vi "calc_phase_map.vi"(3 "noise threshold":dbl=20.0, 4 "u8_ar_image_pixel_array":dbl[][][](array[numeric]), 5 "image name":string="fringe") -> (0 "raw phase map array":dbl[][](array[numeric]), 2 "phase map":T1(plugin-control))   [LabVIEW 2011]
uses:
  global_vars.vi
panel:
  in  "add":dbl
  in  "multi":dbl
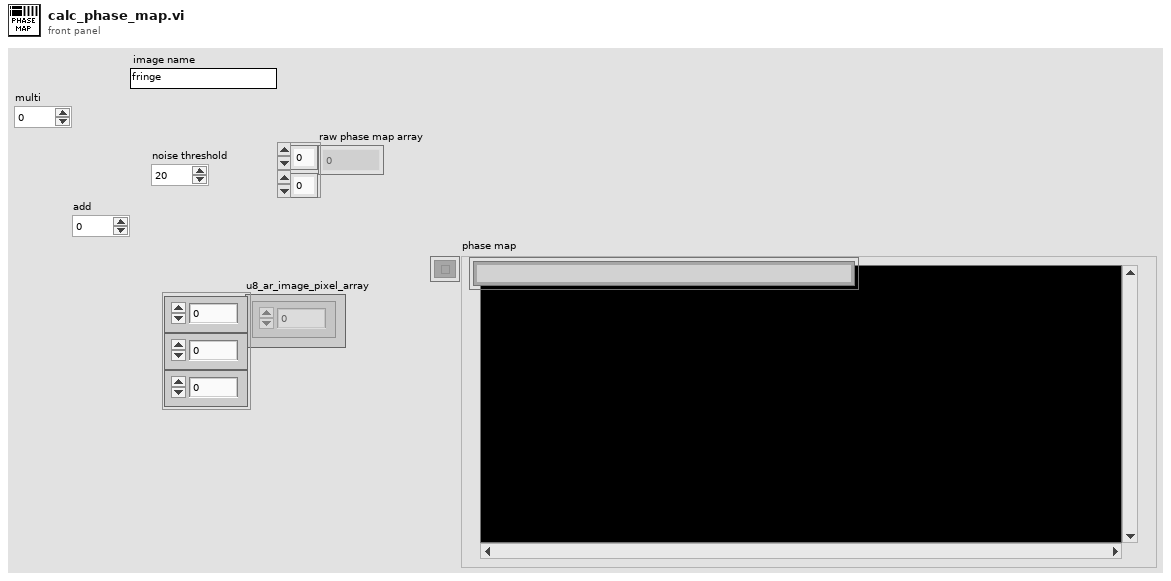
[diagram p1: front panel]
types:
  T1 = typedef "IMAQ Image.ctl" = refnum<image>
  T2 = typedef "Image Type" = u32
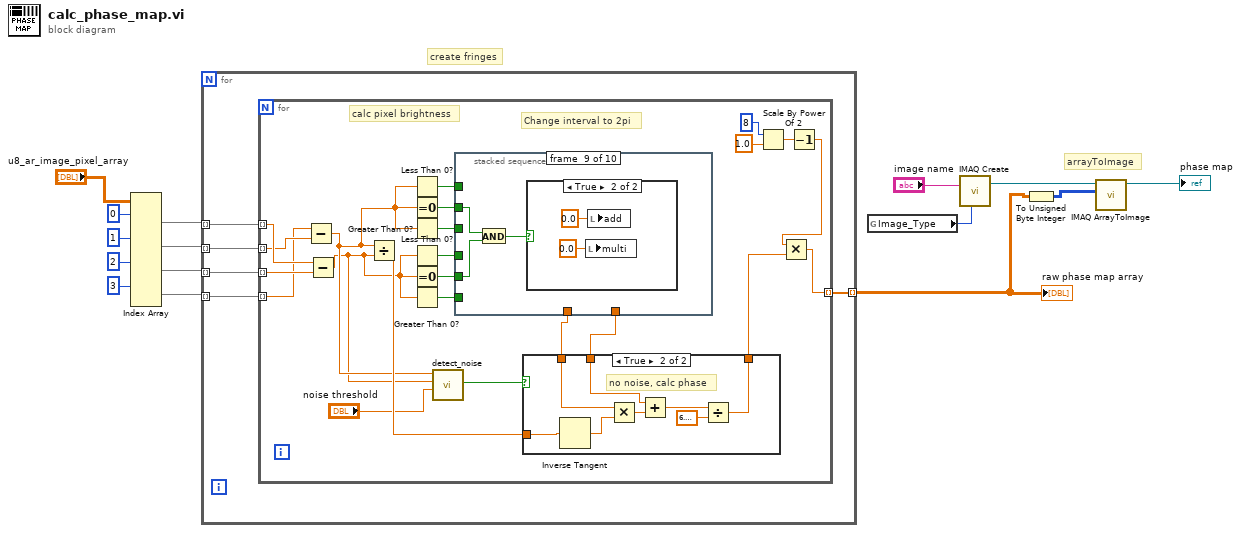
[diagram p0: block diagram]
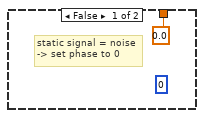
[diagram p2: hidden frame]
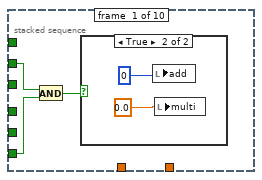
[diagram p3: hidden frame]
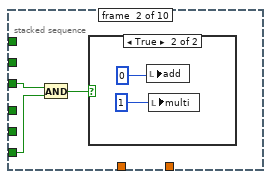
[diagram p5: hidden frame]
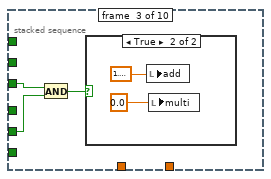
[diagram p7: hidden frame]
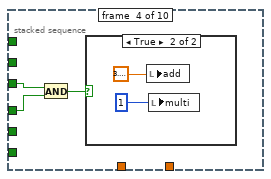
[diagram p9: hidden frame]
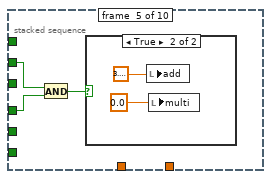
[diagram p11: hidden frame]
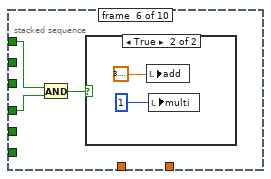
[diagram p13: hidden frame]
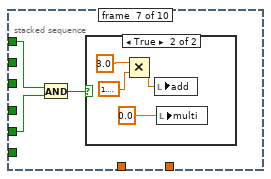
[diagram p15: hidden frame]
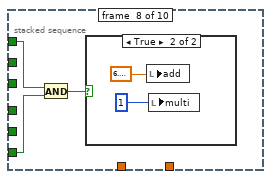
[diagram p17: hidden frame]
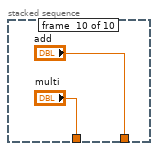
[diagram p20: hidden frame]
diagram:
  # "arrayToImage"
  # "create fringes"
  n1 = Index Array(array="u8_ar_image_pixel_array", index (dim 0) #1=0 ("index (page)"), index (dim 0) #2=1 ("index (page)"), index (dim 0) #3=2 ("index (page)"), index (dim 0) #4=3 ("index (page)")) -> (element #1=w11:dbl[][], element #2=w10:dbl[][], element #3=w9:dbl[][], element #4=w8:dbl[][])  [unwired: 8 in]
  n2 = for {
    tunnel: w11 -> [w20] mode=indexing
    tunnel: w10 -> [w19] mode=indexing
    tunnel: w9 -> [w18] mode=indexing
    tunnel: w8 -> [w17] mode=indexing
    tunnel: [w16] -> w2 mode=indexing
    n3 = for {
      tunnel: w20 -> [w31] mode=indexing
      tunnel: w19 -> [w30] mode=indexing
      tunnel: w18 -> [w27] mode=indexing
      tunnel: w17 -> [w26] mode=indexing
      tunnel: [w39] -> w16 mode=indexing
      # "Change interval to 2pi"
      # "calc pixel brightness"
      n4 = Subtract(x=w26, y=w30) -> (x-y=w23:dbl)
      n5 = Subtract(x=w31, y=w27) -> (x-y=w22:dbl)
      n6 = Divide(x=w23, y=w22) -> (x/y=w25:dbl)
      n7 = Less Than 0?(x=w23) -> (x < 0?=w37:bool)
      n8 = Equal To 0?(x=w23) -> (x = 0?=w36:bool)
      n9 = Greater Than 0?(x=w23) -> (x > 0?=w35:bool)
      n10 = Less Than 0?(x=w22) -> (x < 0?=w32:bool)
      n11 = Equal To 0?(x=w22) -> (x = 0?=w33:bool)
      n12 = Greater Than 0?(x=w22) -> (x > 0?=w34:bool)
      n13 = call "detect_noise.vi"("threshold"="noise threshold", "i1-i3"=w22, "i4-i2"=w23) -> ("is signal"=w24:bool)  [unwired: 7 in, 1 out]
      n14 = stacked-sequence {
        tunnel: w37 -> [_ _ _ _ _ w79 w84 w90 _ _]
        tunnel: w36 -> [w54 _ _ _ w74 _ _ _ w95 _]
        tunnel: w35 -> [_ w59 w63 w69 _ _ _ _ _ _]
        tunnel: w34 -> [w53 w58 _ _ _ _ _ w91 _ _]
        tunnel: w33 -> [_ _ w64 _ _ _ w83 _ w96 _]
        tunnel: w32 -> [_ _ _ w68 w73 w78 _ _ _ _]
        tunnel: [_ _ _ _ _ _ _ _ _ "add"] -> w29
        tunnel: [_ _ _ _ _ _ _ _ _ "multi"] -> w28
        frame #0 {
          n15 = And(x=w54, y=w53) -> (x .and. y?=w55:bool)
          n16 = case shown="True" w55 {
            frame False {
            }
            frame True {
              n17 = local write "add"(0) -> ()
              n18 = local write "multi"(0.0) -> ()
            }
          }
        }
        frame #1 {
          n19 = And(x=w59, y=w58) -> (x .and. y?=w60:bool)
          n20 = case shown="True" w60 {
            frame False {
            }
            frame True {
              n21 = local write "add"(0) -> ()
              n22 = local write "multi"(1) -> ()
            }
          }
        }
        frame #2 {
          n23 = And(x=w63, y=w64) -> (x .and. y?=w65:bool)
          n24 = case shown="True" w65 {
            frame False {
            }
            frame True {
              n25 = local write "add"(1.5707963267948966) -> ()
              n26 = local write "multi"(0.0) -> ()
            }
          }
        }
        frame #3 {
          n27 = And(x=w69, y=w68) -> (x .and. y?=w70:bool)
          n28 = case shown="True" w70 {
            frame False {
            }
            frame True {
              n29 = local write "add"(3.141592653589793) -> ()
              n30 = local write "multi"(1) -> ()
            }
          }
        }
        frame #4 {
          n31 = And(x=w74, y=w73) -> (x .and. y?=w75:bool)
          n32 = case shown="True" w75 {
            frame False {
            }
            frame True {
              n33 = local write "add"(3.141592653589793) -> ()
              n34 = local write "multi"(0.0) -> ()
            }
          }
        }
        frame #5 {
          n35 = And(x=w79, y=w78) -> (x .and. y?=w80:bool)
          n36 = case shown="True" w80 {
            frame False {
            }
            frame True {
              n37 = local write "add"(3.141592653589793) -> ()
              n38 = local write "multi"(1) -> ()
            }
          }
        }
        frame #6 {
          n39 = And(x=w84, y=w83) -> (x .and. y?=w85:bool)
          n40 = case shown="True" w85 {
            frame False {
            }
            frame True {
              n41 = Multiply(x=3.0, y=1.5707963267948966) -> (x*y=w88:dbl)
              n42 = local write "add"(w88) -> ()
              n43 = local write "multi"(0.0) -> ()
            }
          }
        }
        frame #7 {
          n44 = And(x=w90, y=w91) -> (x .and. y?=w92:bool)
          n45 = case shown="True" w92 {
            frame False {
            }
            frame True {
              n46 = local write "add"(6.283185307179586) -> ()
              n47 = local write "multi"(1) -> ()
            }
          }
        }
        frame #8 {
          n48 = And(x=w95, y=w96) -> (x .and. y?=w97:bool)
          n49 = case shown="True" w97 {
            frame False {
            }
            frame True {
              n50 = local write "multi"(0.0 ("multi")) -> ()
              n51 = local write "add"(0.0 ("add")) -> ()
            }
          }
        }
        frame #9 {
        }
      }
      n52 = case shown="True" w24 {
        tunnel: [0.0 w46] -> w40
        tunnel: w29 -> [_ w45]
        tunnel: w28 -> [_ w49]
        tunnel: w25 -> [_ w48]
        frame False {
          (unwired) u8 0
          # "static signal = noise\n-> set phase to 0"
        }
        frame True {
          # "no noise, calc phase"
          n53 = Inverse Tangent(1:w48) -> (0:w47:dbl)
          n54 = Multiply(x=w49, y=w47) -> (x*y=w50:dbl)
          n55 = Add(x=w45, y=w50) -> (x+y=w51:dbl)
          n56 = Divide(x=w51, y=6.283185307179586) -> (x/y=w46:dbl)
        }
      }
      n57 = Scale By Power Of 2(n=8, x=1.0) -> (x*2^n=w42:dbl)
      n58 = Decrement(x=w42) -> (x-1=w41:dbl)
      n59 = Multiply(x=w41, y=w40) -> (x*y=w39:dbl)
    }
  }
  "raw phase map array" <- w2
  n60 = global read "global_vars.vi" "Image_Type"() -> (w3:T2)
  n61 = call "IMAQ Create"("Image Name"="image name", "Image Type"=w3) -> ("New Image"=w4:T1)  [unwired: 2 in, 2 out]
  n62 = To Unsigned Byte Integer(number=w2) -> (unsigned 8bit integer=w1:u8[][])
  n63 = call "IMAQ ArrayToImage"("Image Pixels (U8)"=w1, "Image"=w4) -> ("Image Out"=→"phase map":T1)  [unwired: 8 in, 1 out]
